vi "reset AO_DO_v2.vi"   [LabVIEW 2015]
uses:
  <vilib>/DAQmx/write.llb/DAQmx Write.vi
  <vilib>/DAQmx/write.llb/DAQmx Write (Analog 1D Wfm NChan NSamp).vi
  <vilib>/DAQmx/write.llb/DAQmx Write (Digital 1D Wfm NChan NSamp).vi
  waveforms/usedDOindepofwf.vi
  waveforms/usedAOindepofwf.vi
  Objects/2pparameters.vi
  Objects/waveformsAObuffer.vi
  Objects/waveformsDObuffer.vi
  <vilib>/Waveform/DWDTOps.llb/DWDT Analog to Digital.vi
  <vilib>/DAQmx/configure/timing.llb/DAQmx Timing (Sample Clock).vi
  <vilib>/Waveform/DWDTOps.llb/DWDT Uncompress Digital.vi
  <vilib>/DAQmx/miscellaneous.llb/DAQmx Fill In Error Info.vi
  <resource>/objmgr/daqmx.rc
types:
  T1 = cluster{"StageS":i32, "StageL":i32, "currmeas data dir":path, "image OD":u16, "contour OD":u16, "point OD":u16, "AOlines":tag[], "AIlines":tag[], "CI lines":tag[], "DO lines":tag[], "AO names":string[], "CI names":string[], "AI names":string[], "DO names":string[], "CIextensions":string[], "AIextensions":string[], "Voltage to Ygalvo":i32, "Voltage to Xgalvo":i32, "Voltage to patch":i32, "640 shutter":i32, "2P shutter":i32, "LT timestamp":u32, "Vp":i32, "Ip":i32, "camera trigger":i32, "master data dir":path}
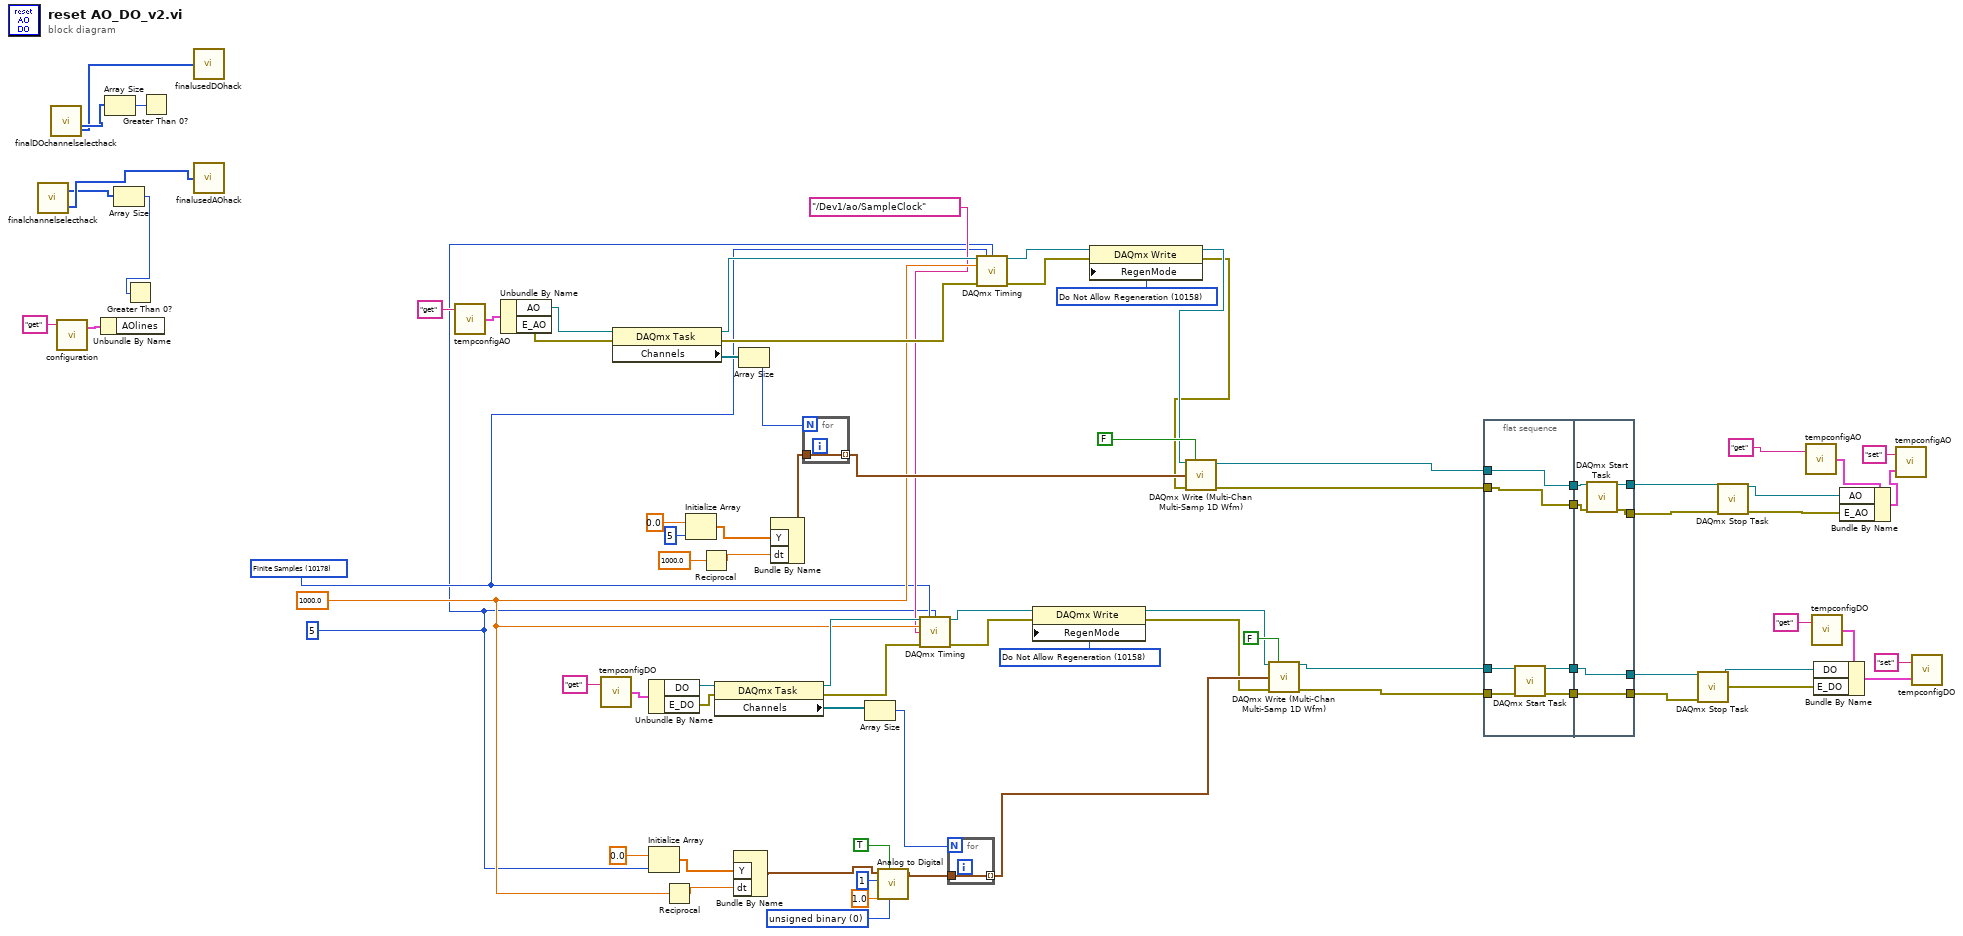
[diagram p0: block diagram]
diagram:
  w15 = 10158 items=["Allow Regeneration"=10097, "Do Not Allow Regeneration"=10158] ("RegenMode")
  w38 = 10158 items=["Allow Regeneration"=10097, "Do Not Allow Regeneration"=10158] ("RegenMode")
  w9 = 10178 items=["Finite Samples"=10178, "Continuous Samples"=10123, "Hardware Timed Single Point"=12522] ("sample mode")
  w8 = 5 ("dimension size")
  w11 = 1000.0 ("dt")
  w55 = u16 0 items=["unsigned binary", "offset binary", "2's complement"] ("data format (offset binary)")
  n1 = call "finalchannelselecthack.vi"() -> ("usedAO sorted"=w73:u32[], "presorted indices"=w74:u32[])  [unwired: 1 in]
  n2 = call "finalDOchannelselecthack.vi"() -> ("usedDO"=w72:u32[], "presorted indices"=w63:u32[])  [unwired: 1 in]
  n3 = call "configuration.vi"("command"="get") -> ("config out"=w76:T1)  [unwired: 2 in, 1 out]
  n4 = Unbundle By Name(w76) -> ()  [unwired: 1 out]
  n5 = Array Size(array=w72) -> (size(s)=w71:i32)
  n6 = Array Size(array=w73) -> (size(s)=w75:i32)
  n7 = Greater Than 0?(x=w75) -> ()  [unwired: 1 out]
  n8 = Greater Than 0?(x=w71) -> ()  [unwired: 1 out]
  n9 = call "finalusedDOhack.vi"("presorted indices"=w63) -> ()  [unwired: 1 out]
  n10 = call "finalusedAOhack.vi"("presorted indices"=w74) -> ()  [unwired: 1 out]
  n11 = call "tempconfigAO.vi"("command"="get") -> ("Temp Config out"=w21:cluster{"AO":refnum<k21>, "E_AO":errorcluster})  [unwired: 1 in]
  n12 = Unbundle By Name(w21) -> ("AO"=w20:refnum<k21>, "E_AO"=w19:errorcluster)
  n13 = call "tempconfigDO.vi"("command"="get") -> ("Temp Config out"=w61:cluster{"DO":refnum<k21>, "E_DO":errorcluster})  [unwired: 1 in]
  n14 = property class="DAQmx Task"(reference=w20, error in=w19) -> (reference out=w13:refnum<k21>, error out=w12:errorcluster, "Channels"=w78:refnum<k21>[])
  n15 = Unbundle By Name(w61) -> ("DO"=w60:refnum<k21>, "E_DO"=w59:errorcluster)
  n16 = Initialize Array(0.0 ("element"), w8) -> (w52:dbl[])
  n17 = Reciprocal(x=w11) -> (1/x=w54:dbl)
  n18 = Initialize Array(0.0 ("element"), 5 ("dimension size")) -> (w47:dbl[])
  n19 = Reciprocal(x=1000.0 ("dt")) -> (1/x=w43:dbl)
  n20 = property class="DAQmx Task"(reference=w60, error in=w59) -> (reference out=w42:refnum<k21>, error out=w41:errorcluster, "Channels"=w80:refnum<k21>[])
  n21 = Bundle By Name("Y"=w52, "dt"=w54) -> (w51:waveform(dbl))  [unwired: 1 in]
  n22 = Array Size(array=w78) -> (size(s)=w17:i32)
  n23 = Bundle By Name("Y"=w47, "dt"=w43) -> (w18:waveform(dbl))  [unwired: 1 in]
  n24 = for {
    N: w17 -> [_]
    tunnel: [w82] -> w16 mode=indexing
    tunnel: w18 -> [w82]
  }
  n25 = Array Size(array=w80) -> (size(s)=w50:i32)
  n26 = call-poly <vilib>:"Analog to Digital.vi"("data format (offset binary)"=w55, "compress digital (T)"=TRUE, "full-scale range (pk-pk)"=1.0, "resolution (16 bit)"=1, "analog waveform"=w51) -> ("digital waveform"=w49:digitalwaveform)  [unwired: 3 in, 3 out]
  n27 = call-poly <vilib>:"DAQmx Timing.vi"("task/channels in"=w42, "sample mode"=w9, "samples per channel"=w8, "rate"=w11, "source"=tag "/Dev1/ao/SampleClock", "error in"=w41) -> ("task out"=w40:refnum<k21>, "error out"=w39:errorcluster)  [unwired: 8 in]
  n28 = for {
    N: w50 -> [_]
    tunnel: [w83] -> w48 mode=indexing
    tunnel: w49 -> [w83]
  }
  n29 = call-poly <vilib>:"DAQmx Timing.vi"("task/channels in"=w13, "sample mode"=w9, "samples per channel"=w8, "rate"=w11, "error in"=w12) -> ("task out"=w7:refnum<k21>, "error out"=w14:errorcluster)  [unwired: 9 in]
  n30 = property class="DAQmx Write"(reference=w40, error in=w39, "RegenMode"=w38) -> (reference out=w36:refnum<k21>, error out=w37:errorcluster)
  n31 = property class="DAQmx Write"(reference=w7, error in=w14, "RegenMode"=w15) -> (reference out=w6:refnum<k21>, error out=w5:errorcluster)
  n32 = call-poly "DAQmx Write (Multi-Chan Multi-Samp 1D Wfm).vi"("task/channels in"=w6, "auto start"=FALSE, "data"=w16, "error in"=w5) -> ("task out"=w4:refnum<k21>, "error out"=w3:errorcluster)  [unwired: 9 in, 1 out]
  n33 = call-poly "DAQmx Write (Multi-Chan Multi-Samp 1D Wfm).vi"("task/channels in"=w36, "auto start"=FALSE, "data"=w48, "error in"=w37) -> ("task out"=w2:refnum<k21>, "error out"=w1:errorcluster)  [unwired: 9 in, 1 out]
  n34 = flat-sequence {
    tunnel: w2 -> [w89]
    tunnel: w1 -> [w88]
    tunnel: w4 -> [w87]
    tunnel: [w87] -> w35
    tunnel: w3 -> [w86]
    tunnel: [w86] -> w34
    tunnel: [w85] -> w30
    tunnel: [w84] -> w28
    tunnel: w35 -> [w95]
    tunnel: w34 -> [w94]
    tunnel: [w93] -> w33
    tunnel: [w92] -> w32
    tunnel: [w91] -> w31
    tunnel: w30 -> [w91]
    tunnel: [w90] -> w29
    tunnel: w28 -> [w90]
    frame #0 {
      n35 = call <vilib>:"DAQmx Start Task.vi"("task/channels in"=w89, "error in"=w88) -> ("task out"=w85:refnum<k21>, "error out"=w84:errorcluster)  [unwired: 12 in]
    }
    frame #1 {
      n36 = call <vilib>:"DAQmx Start Task.vi"("task/channels in"=w95, "error in"=w94) -> ("task out"=w93:refnum<k21>, "error out"=w92:errorcluster)  [unwired: 12 in]
    }
  }
  n37 = call <vilib>:"DAQmx Stop Task.vi"("task/channels in"=w31, "error in"=w29) -> ("task out"=w27:refnum<k21>, "error out"=w26:errorcluster)  [unwired: 12 in]
  n38 = call <vilib>:"DAQmx Stop Task.vi"("task/channels in"=w33, "error in"=w32) -> ("task out"=w25:refnum<k21>, "error out"=w24:errorcluster)  [unwired: 12 in]
  n39 = call "tempconfigAO.vi"("command"="get") -> ("Temp Config out"=w65:cluster{"AO":refnum<k21>, "E_AO":errorcluster})  [unwired: 1 in]
  n40 = call "tempconfigDO.vi"("command"="get") -> ("Temp Config out"=w68:cluster{"DO":refnum<k21>, "E_DO":errorcluster})  [unwired: 1 in]
  n41 = Bundle By Name(cluster=w68, "DO"=w27, "E_DO"=w26) -> (w70:cluster{"DO":refnum<k21>, "E_DO":errorcluster})
  n42 = Bundle By Name(cluster=w65, "AO"=w25, "E_AO"=w24) -> (w66:cluster{"AO":refnum<k21>, "E_AO":errorcluster})
  n43 = call "tempconfigAO.vi"("Temp Config in"=w66, "command"="set") -> ()  [unwired: 1 out]
  n44 = call "tempconfigDO.vi"("Temp Config in"=w70, "command"="set") -> ()  [unwired: 1 out]
